vi "CaseStructure-Ver1.vi"() -> ()   [LabVIEW 2018]
panel:
  in  "Boolean":bool
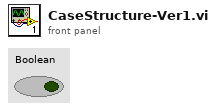
[diagram p1: front panel]
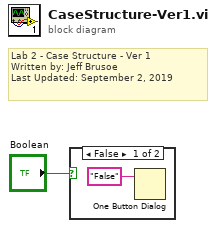
[diagram p0: block diagram]
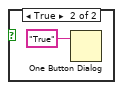
[diagram p2: hidden frame]
diagram:
  # "Lab 2 - Case Structure - Ver 1\nWritten by: Jeff Brusoe\nLast Updated: September 2, 2019"
  n1 = case shown="False" "Boolean" {
    frame False {
      n2 = One Button Dialog(message="False") -> ()  [unwired: 1 in, 1 out]
    }
    frame True {
      n3 = One Button Dialog(message="True") -> ()  [unwired: 1 in, 1 out]
    }
  }
